vi "Environments.vi"(8 "Error In":errorcluster, 11 "Environments in":T1) -> (0 "Error Out":errorcluster, 3 "Environments out":T1)   [LabVIEW 2018]
uses:
  Environments.ctl
panel:
  out "Temperature Max":dbl=21.0 caption="Numeric" format="%.1f"
  out "Humidity Max":dbl=21.0 caption="Numeric" format="%.1f"
  out "Pressure Max":dbl=21.0 caption="Numeric" format="%.1f"
  out "Temperature Min":dbl=21.0 caption="Numeric" format="%.1f"
  out "Humidity Min":dbl=21.0 caption="Numeric" format="%.1f"
  out "Pressure Min":dbl=21.0 caption="Numeric" format="%.1f"
  in  "Temperature":dbl=21.0 caption="Numeric" min=0.0 max=100.0 format="%.1f"
  in  "Humidity":dbl=21.0 caption="Numeric" min=0.0 max=100.0 format="%.1f"
  in  "Pressure":dbl=21.0 caption="Numeric" min=0.0 max=1000.0 format="%.1f"
  in  "Save":bool
  # "Enviroment:"
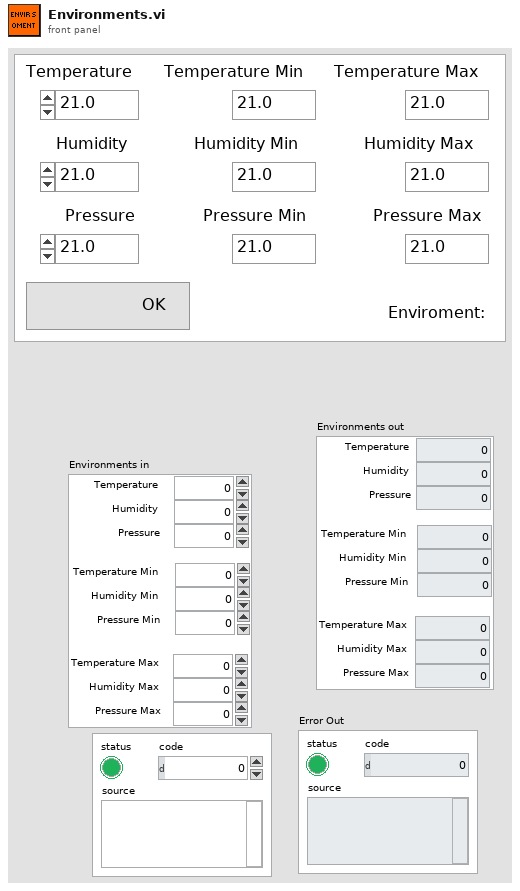
[diagram p1: front panel]
types:
  T1 = typedef "Environments.ctl" = cluster{"Temperature Min":dbl, "Humidity Min":dbl, "Pressure Min":dbl, "Temperature Max":dbl, "Humidity Max":dbl, "Pressure Max":dbl, "Temperature":dbl, "Humidity":dbl, "Pressure":dbl}
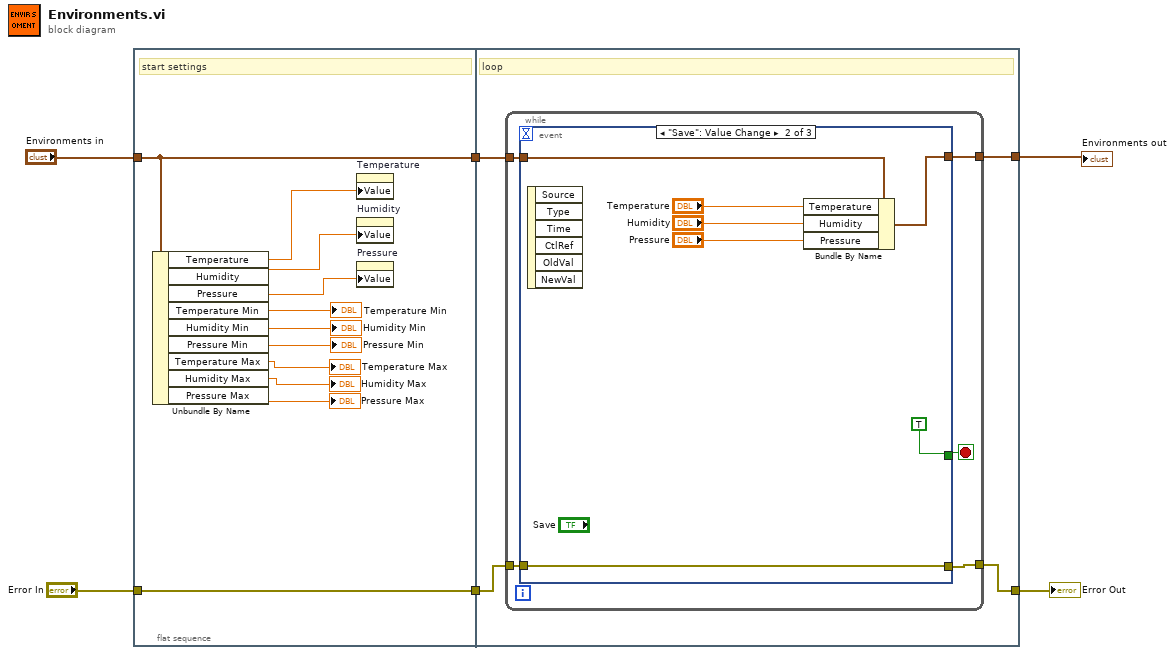
[diagram p0: block diagram]
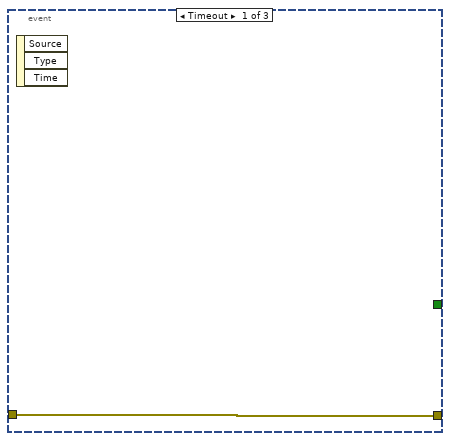
[diagram p2: hidden frame]
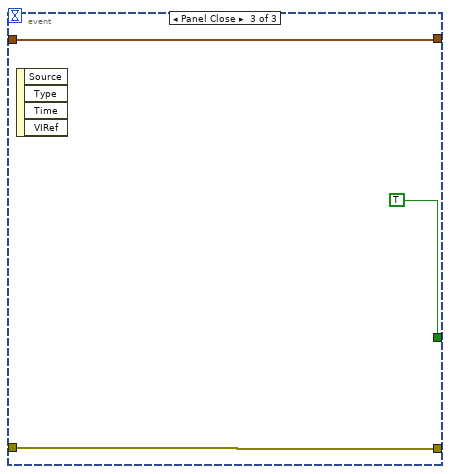
[diagram p3: hidden frame]
diagram:
  n1 = flat-sequence {
    tunnel: [w17] -> w6
    tunnel: "Environments in" -> [w17]
    tunnel: [w16] -> w5
    tunnel: "Error In" -> [w16]
    tunnel: w6 -> [w21]
    tunnel: [w20] -> w2
    tunnel: w5 -> [w18]
    tunnel: [w19] -> w3
    frame #0 {
      # "start settings"
      n2 = Unbundle By Name(w17) -> ("Temperature"=w7:dbl, "Humidity"=w15:dbl, "Pressure"=w14:dbl, "Temperature Min"=→"Temperature Min":dbl, "Humidity Min"=→"Humidity Min":dbl, "Pressure Min"=→"Pressure Min":dbl, "Temperature Max"=→"Temperature Max":dbl, "Humidity Max"=→"Humidity Max":dbl, "Pressure Max"=→"Pressure Max":dbl)
      n3 = property on="Temperature" class="DigNum (strict)"("Value"=w7) -> ()  [unwired: 2 in, 2 out]
      n4 = property on="Humidity" class="DigNum (strict)"("Value"=w15) -> ()  [unwired: 2 in, 2 out]
      n5 = property on="Pressure" class="DigNum (strict)"("Value"=w14) -> ()  [unwired: 2 in, 2 out]
    }
    frame #1 {
      # "loop"
      n6 = while {
        tunnel: w21 -> [w25]
        tunnel: [w24] -> w20
        tunnel: [w23] -> w19
        tunnel: w18 -> [w22]
        stop <- w26 stop-if-true
        n7 = event shown="[1] \"Save\": Value Change" {
          selector: _ -> [_ _ _]
          dyn-events: _ -> [_ _ _]
          timeout: _ -> [_ _ _]
          tunnel: [_ TRUE TRUE] -> w26
          tunnel: w25 -> [_ w33 w36]
          tunnel: [_ w32 w36] -> w24
          tunnel: [w27 w31 w35] -> w23
          tunnel: w22 -> [w27 w31 w35]
          event Timeout {
            n8 = event-data() -> ()  [unwired: 1 in, 3 out]
          }
          event "Save": Value Change {
            n9 = event-data() -> ()  [unwired: 1 in, 6 out]
            n10 = Bundle By Name(cluster=w33, "Temperature"="Temperature", "Humidity"="Humidity", "Pressure"="Pressure") -> (w32:T1)
          }
          event Panel Close {
            n11 = event-data() -> ()  [unwired: 1 in, 4 out]
          }
        }
      }
    }
  }
  "Error Out" <- w3
  "Environments out" <- w2
